vi "Window Element String To Enum.vi"(8 "Error In":errorcluster, 11 "Window Element Str":string) -> (0 "Error Out":errorcluster, 3 "Window Element":T1)   [LabVIEW 2021, in "Appearance Actor.lvlib" / "Generic Theme.lvclass"]
uses:
  Generic Theme.lvclass
  Typedefs/Window Element--enum.ctl
  Generic Theme.lvclass/Generic Theme.ctl
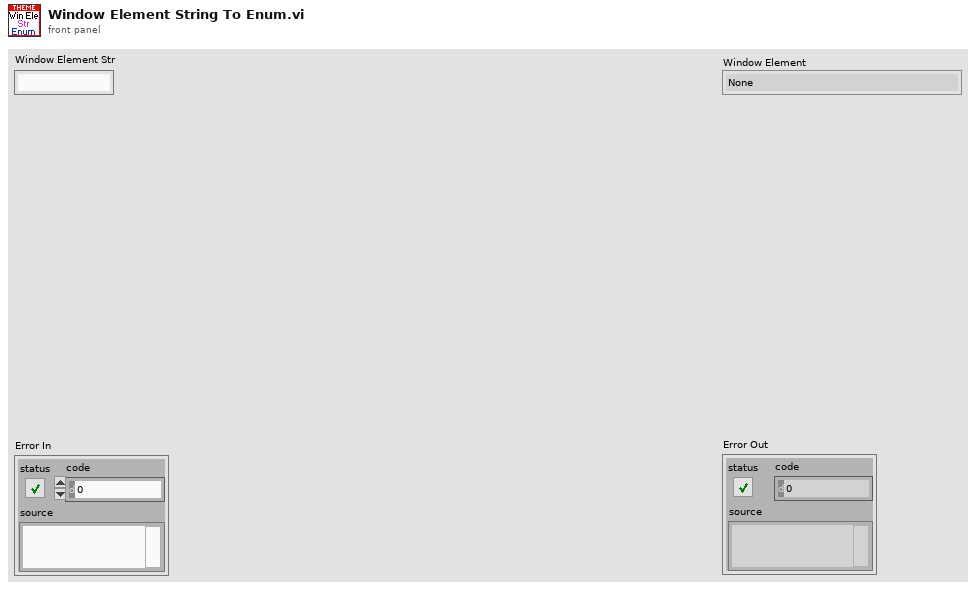
[diagram p1: front panel]
types:
  T1 = typedef "Appearance Actor.lvlib/Generic Theme.lvclass/Window Element--enum.ctl" = enum16{"None", "TB", "SM", "BP", "SB"}
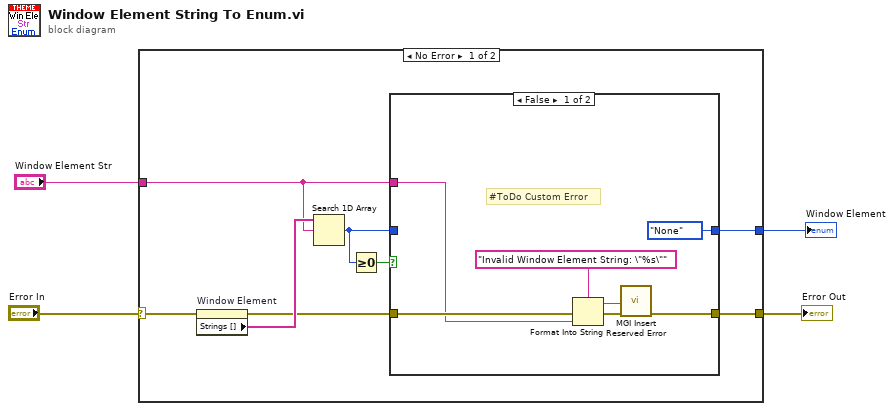
[diagram p0: block diagram]
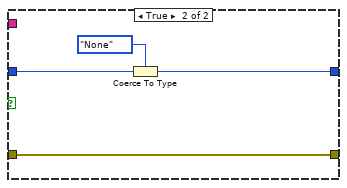
[diagram p2: hidden frame]
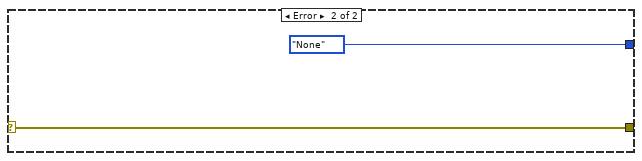
[diagram p3: hidden frame]
diagram:
  n1 = case shown="No Error" "Error In" {
    selector: "Error In" -> [w12 w25]
    tunnel: [w6 w25] -> w3
    tunnel: "Window Element Str" -> [w5 _]
    tunnel: [w8 Window_Element--enum."None" ("Window Element")] -> w1
    frame No Error {
      n2 = property on="Window Element" class="Enum (strict)"(error in=w12) -> (error out=w7:errorcluster, "Strings []"=w11:string[])  [unwired: 1 in, 1 out]
      n3 = Search 1D Array(1D array=w11, element=w5) -> (index of element=w9:i32)  [unwired: 1 in]
      n4 = Greater Or Equal To 0?(x=w9) -> (x >= 0?=w10:bool)
      n5 = case shown="False" w10 {
        tunnel: w9 -> [_ w23]
        tunnel: [Window_Element--enum."None" ("Window Element") w21] -> w8
        tunnel: w7 -> [w19 w20]
        tunnel: [w18 w20] -> w6
        tunnel: w5 -> [w16 _]
        frame False {
          # "#ToDo Custom Error"
          n6 = Format Into String(format string="Invalid Window Element String: \"%s\"", error in=w19, w16) -> (resulting string=w14:string, error out=w17:errorcluster)  [unwired: 1 in]
          n7 = call <userlib>:"MGI Insert Reserved Error.vi"("Error In"=w17, "Error Description"=w14) -> ("Error Out"=w18:errorcluster)  [unwired: 9 in]
        }
        frame True {
          n8 = Coerce To Type(0:w23, 1:Window_Element--enum."None" ("Window Element")) -> (2:w21:T1)
        }
      }
    }
    frame Error {
    }
  }
  "Window Element" <- w1
  "Error Out" <- w3
